vi "Wave2D_Solver.vi"(0 "F(t, x, y)":dbl[][][](array[numeric]), 1 "Initial Value":dbl[][](array[numeric]), 2 "Initial Derivative":dbl[][](array[numeric]), 5 "k":dbl=1.0, 7 "a":dbl, 9 "Domain":T2={"t"={"initial t"=0.0, "final t"=1.0, "# of t-points"=11}, "x"={"start x"=0.0, "end x"=1.0, "# of x-points"=11}, "y"={"start y"=0.0, "end y"=1.0, "# of y-points"=11}}, 11 "error in (no error)":errorcluster, 12 "Boundary Condition":cluster{"type":T1, "Value":dbl[][]}[](array[cluster]) {"type" items=["Dirichlet", "Neumann"]}) -> (4 "U(t, x, y)":dbl[][][](array[numeric]), 15 "error out":errorcluster)   [LabVIEW 2020, in "NI_PDE.lvlib"]
uses:
  <vilib>/gmath/NI_PDE.lvlib
  <vilib>/gmath/pde.llb/Common/PDE_BC Type.ctl
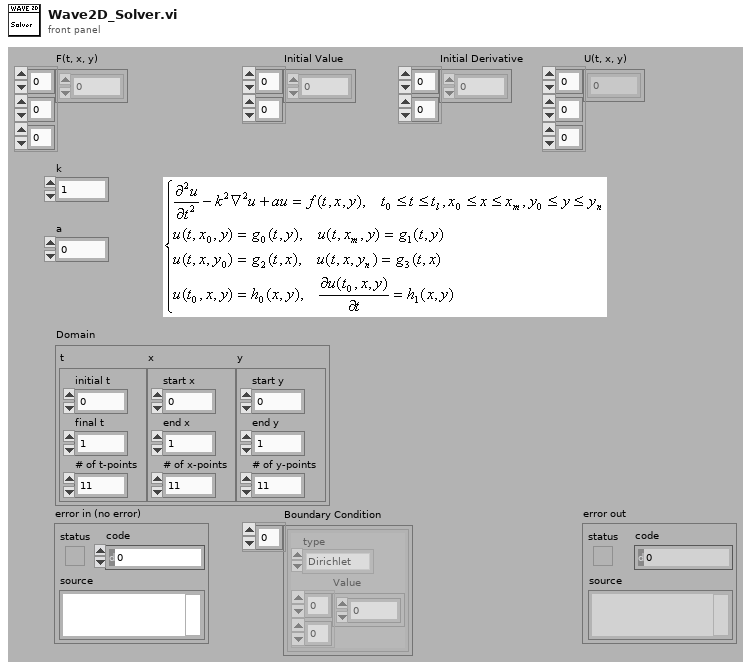
[diagram p1: front panel]
types:
  T1 = typedef "NI_PDE.lvlib/PDE_BC Type.ctl" = i32
  T2 = cluster{"t":cluster{"initial t":dbl, "final t":dbl, "# of t-points":i32}, "x":cluster{"start x":dbl, "end x":dbl, "# of x-points":i32}, "y":cluster{"start y":dbl, "end y":dbl, "# of y-points":i32}}
  T3 = typedef "NI_PDE.lvlib/Wave2D_Data.ctl" = cluster{"PDE":cluster{"k":dbl, "a":dbl, "F(t, x, y)":dbl[][][]}, "Domain":cluster{"t":cluster{"initial t":dbl, "final t":dbl, "# of t-points":i32}, "x":cluster{"start x":dbl, "end x":dbl, "# of x-points":i32}, "y":cluster{"start y":dbl, "end y":dbl, "# of y-points":i32}, "delta":cluster{"delta t":dbl, "delta x":dbl, "delta y":dbl}}, "BC":cluster{"Start X":cluster{"type":T1, "Value":dbl[][]}, "End X":cluster{"type":T1, "Value":dbl[][]}, "Start Y":cluster{"type":T1, "Value":dbl[][]}, "End Y":cluster{"type":T1, "Value":dbl[][]}}, "Corner":cluster{"Start X & Start Y":dbl[], "Start X & End Y":dbl[], "End X & Start Y":dbl[], "End X & End Y":dbl[]}, "IC":cluster{"Value":dbl[][], "Derivative":dbl[][]}, "P":cluster{"Sub Diag":dbl[], "Diag":dbl[], "Super Diag":dbl[], "P":T4}, "LU of P":cluster{"L":dbl[], "U":cluster{"Diag":dbl[], "Super Diag":dbl[], "2nd Super Diag":dbl[]}, "Pivot":i32[]}, "Q":cluster{"Sub Diag":dbl[], "Diag":dbl[], "Super Diag":dbl[], "Q":T4}, "LU of Q":cluster{"L":dbl[], "U":cluster{"Diag":dbl[], "Super Diag":dbl[], "2nd Super Diag":dbl[]}, "Pivot":i32[]}, "State":cluster{"U":dbl[][], "Old U":dbl[][], "V&W":dbl[][], "x start index":i32, "x length":i32, "y start index":i32, "y length":i32}}
  T4 = typedef "NI_Matrix.lvlib/RealMatrix.ctl" = dbl[][]
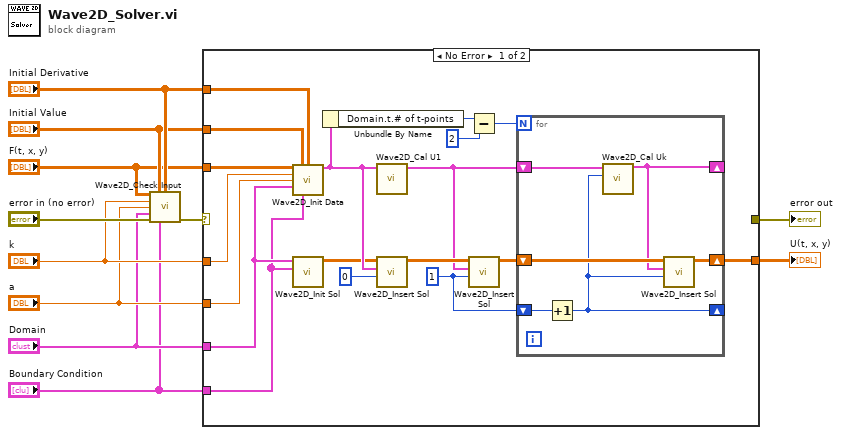
[diagram p0: block diagram]
diagram:
  n1 = call <vilib>:"Wave2D_Check Input.vi"("F(t, x, y)"="F(t, x, y)", "Initial Value"="Initial Value", "Initial Derivative"="Initial Derivative", "k"="k", "a"="a", "Domain"="Domain", "error in (no error)"="error in (no error)", "Boundary Condition"="Boundary Condition") -> ("error out"=w10:errorcluster)  [unwired: 7 out]
  n2 = case shown="No Error" w10 {
    selector: w10 -> [_ w36]
    tunnel: [_ w36] -> w9
    tunnel: "Initial Derivative" -> [w27 _]
    tunnel: "Initial Value" -> [w28 _]
    tunnel: "F(t, x, y)" -> [w29 _]
    tunnel: "k" -> [w26 _]
    tunnel: "a" -> [w25 _]
    tunnel: "Domain" -> [w21 _]
    tunnel: "Boundary Condition" -> [w20 _]
    tunnel: [w12 _] -> w1
    frame No Error {
      w13 = 1 ("time step")
      n3 = call <vilib>:"Wave2D_Init Data.vi"("F(t, x, y)"=w29, "Initial Value"=w28, "Initial Derivative"=w27, "k"=w26, "a"=w25, "Domain"=w21, "Boundary Condition"=w20) -> ("Wave2D Data"=w19:T3)  [unwired: 8 out]
      n4 = call <vilib>:"Wave2D_Init Sol.vi"("Boundary Condition"=w20, "Domain"=w21) -> ("U(t, x, y)"=w18:dbl[][][])  [unwired: 9 out]
      n5 = Unbundle By Name(w19) -> ("Domain.t.# of t-points"=w24:i32)
      n6 = call <vilib>:"Wave2D_Cal U1.vi"("Wave2D Data In"=w19) -> ("Wave2D Data Out"=w15:T3)  [unwired: 10 out]
      n7 = call <vilib>:"Wave2D_Insert Sol.vi"("time step"=0, "Wave2D Data"=w19, "U(t, x, y) In"=w18) -> ("U(t, x, y) Out"=w16:dbl[][][])  [unwired: 8 out]
      n8 = Subtract(x=w24, y=2) -> (x-y=w23:i32)
      n9 = call <vilib>:"Wave2D_Insert Sol.vi"("time step"=w13, "Wave2D Data"=w15, "U(t, x, y) In"=w16) -> ("U(t, x, y) Out"=w14:dbl[][][])  [unwired: 8 out]
      n10 = for {
        N: w23 -> [_]
        shift-right: [w32] -> _
        shift-left: w15 -> [w35]
        shift-right: [w33] -> w12
        shift-left: w14 -> [w34]
        shift-right: [w30] -> _
        shift-left: w13 -> [w31]
        n11 = Increment(x=w31) -> (x+1=w30:i32)
        n12 = call <vilib>:"Wave2D_Cal Uk.vi"("time step"=w30, "Wave2D Data In"=w35) -> ("Wave2D Data Out"=w32:T3)  [unwired: 9 out]
        n13 = call <vilib>:"Wave2D_Insert Sol.vi"("time step"=w30, "Wave2D Data"=w32, "U(t, x, y) In"=w34) -> ("U(t, x, y) Out"=w33:dbl[][][])  [unwired: 8 out]
      }
    }
    frame Error {
    }
  }
  "U(t, x, y)" <- w1
  "error out" <- w9
